vi "ELVIS III v1.1 Start AI Continuous.vi"(4 "Minimum (S/s)":dbl=1000.0, 5 "Sample Rate":dbl=1000.0 min=1000.0 max=1000000.0, 6 "Maximum (S/s)":dbl=1000000.0, 7 "Scaling Constants List":T1, 8 "error in (no error)":errorcluster, 10 "AI (Continuous) Channels List":T3, 11 "AI (Continuous) Ref In":T5) -> (0 "error out":errorcluster, 3 "AI (Continuous) Ref Out":T5)   [LabVIEW 2021]
uses:
  <vilib>/myRIO/Common/Instrument Driver Framework/Utilities/typedefs/myRIO v1.0 Reference.ctl
  <vilib>/myRIO/Common/Instrument Driver Framework/Utilities/typedefs/Generic FPGA Reference.ctl
  <vilib>/myRIO/Common/Instrument Driver Framework/ELVIS III v1.0/AI Continuous/typedefs/AI Continuous Channels List.ctl
  <vilib>/myRIO/Common/Instrument Driver Framework/ELVIS III v1.0/AI Continuous/typedefs/ELVIS III v1.0 AI Continuous Channels Enum.ctl
  <vilib>/myRIO/Common/Instrument Driver Framework/Utilities/typedefs/Analog Scaling Constants List.ctl
  <vilib>/myRIO/Common/Instrument Driver Framework/Utilities/typedefs/Analog Scaling Constants.ctl
  <vilib>/myRIO/Common/Instrument Driver Framework/ELVIS III v1.0/AI Block/typedefs/ELVIS III AI Block Channels FPGA Reference.ctl
  <vilib>/rvi/errors/niLvFpgaAdjustHostInterfaceError.vi
  <vilib>/rvi/interface/nirviReadWriteControl/nirviReadWriteControl.xnode
  <vilib>/rvi/interface/nirviMethod/nirviMethod.xnode
  <vilib>/rvi/errors/niLvFpgaMergeErrorWithErrorCode.vi
  <vilib>/rvi/interface/Simulation/niFpgaSimulationCallBeginRW.vi
  <vilib>/FPGAPlugInAG/Dynamic/niLvFpga_StartFifo_Dynamic.vi
  <vilib>/FPGAPlugInAG/Dynamic/niLvFpga_StopFifo_Dynamic.vi
  NiFpgaLv.dll
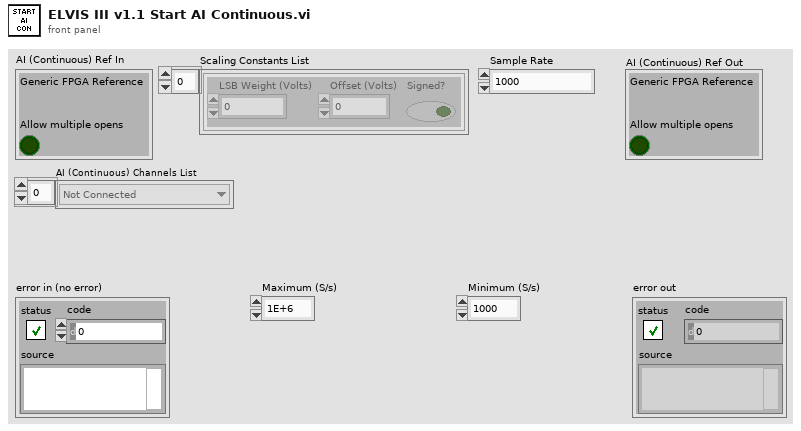
[diagram p1: front panel]
types:
  T1 = typedef "Analog Scaling Constants List.ctl" = T2[]
  T2 = typedef "Analog Scaling Constants.ctl" = cluster{"LSB Weight (Volts)":dbl, "Offset (Volts)":dbl, "Signed?":bool}
  T3 = typedef "AI Continuous Channels List.ctl" = T4[]
  T4 = typedef "ELVIS III v1.0 AI Continuous Channels Enum.ctl" = enum16{"Not Connected", "A/AI0 (Continuous)", "A/AI1 (Continuous)", "A/AI2 (Continuous)", "A/AI3 (Continuous)", "A/AI4 (Continuous)", "A/AI5 (Continuous)", "A/AI6 (Continuous)", "A/AI7 (Continuous)", "A/AI0 (DIFF Continuous)", "A/AI1 (DIFF Continuous)", "A/AI2 (DIFF Continuous)", "A/AI3 (DIFF Continuous)", "B/AI0 (Continuous)", "B/AI1 (Continuous)", "B/AI2 (Continuous)", "B/AI3 (Continuous)", "B/AI4 (Continuous)", "B/AI5 (Continuous)", "B/AI6 (Continuous)", "B/AI7 (Continuous)", "B/AI0 (DIFF Continuous)", "B/AI1 (DIFF Continuous)", "B/AI2 (DIFF Continuous)", "B/AI3 (DIFF Continuous)"}
  T5 = typedef "myRIO v1.0 Reference.ctl" = cluster{"Generic FPGA Reference":T6, "Allow multiple opens":bool}
  T6 = typedef "Generic FPGA Reference.ctl" = refnum<k20>
  T7 = typedef "ELVIS III AI Block Channels FPGA Reference.ctl" = refnum<k20>
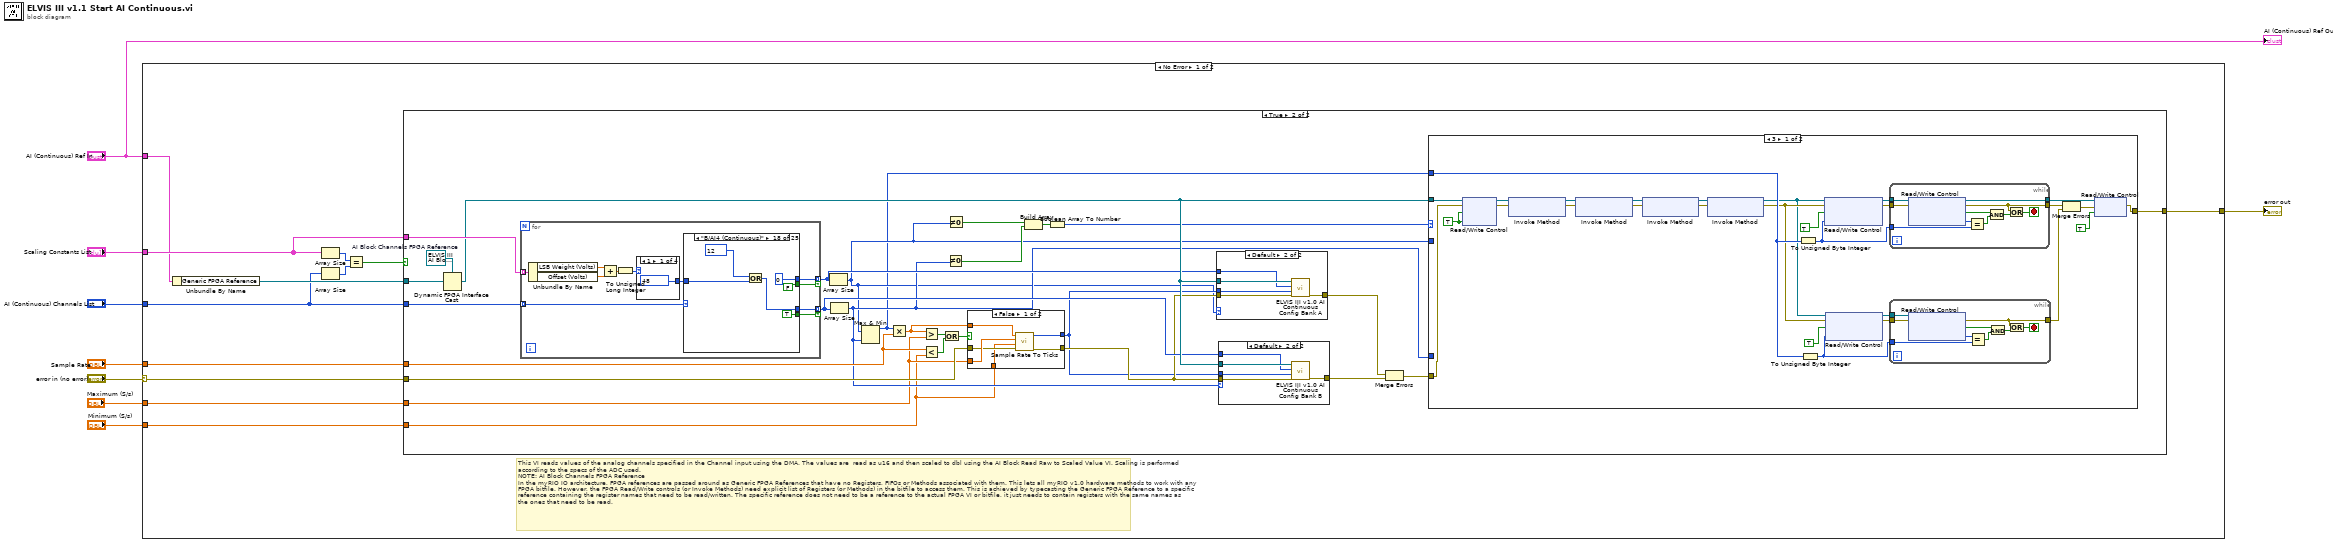
[diagram p0: block diagram]
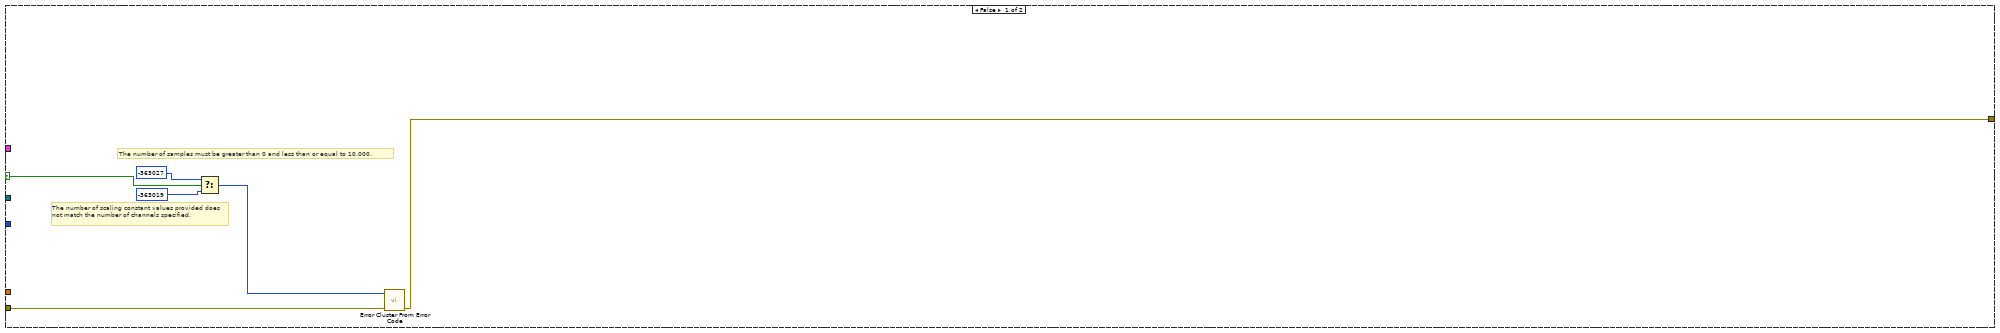
[diagram p2: hidden frame]
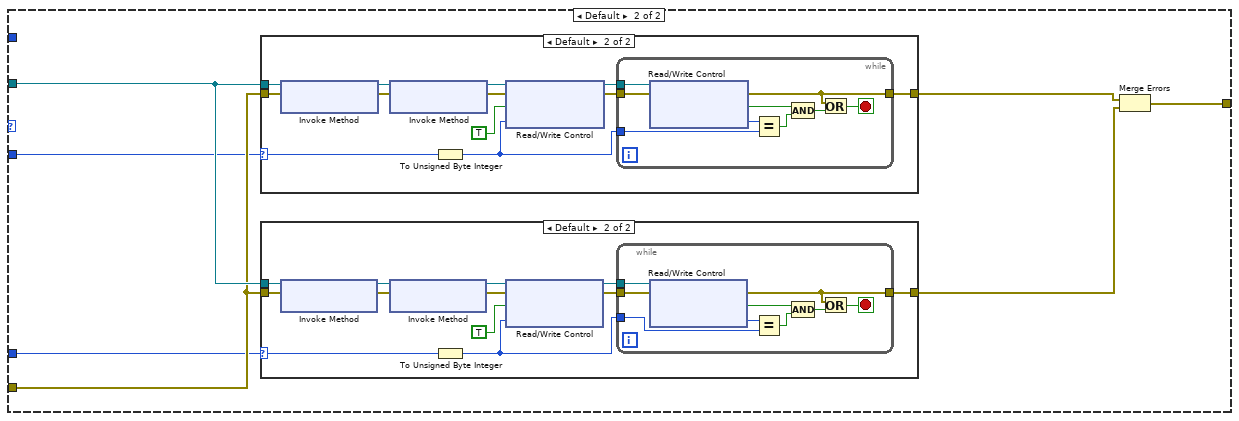
[diagram p3: hidden frame]
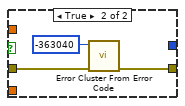
[diagram p6: hidden frame]
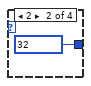
[diagram p7: hidden frame]
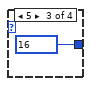
[diagram p8: hidden frame]
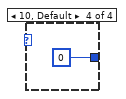
[diagram p9: hidden frame]
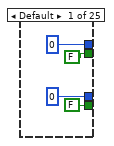
[diagram p10: hidden frame]
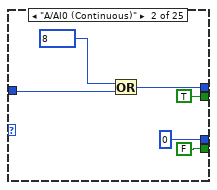
[diagram p11: hidden frame]
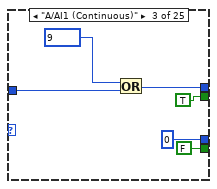
[diagram p12: hidden frame]
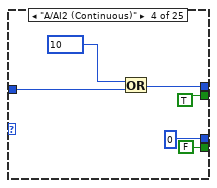
[diagram p13: hidden frame]
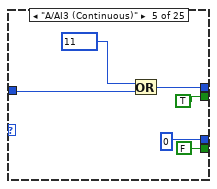
[diagram p14: hidden frame]
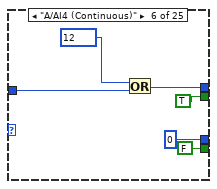
[diagram p15: hidden frame]
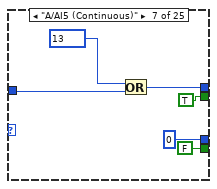
[diagram p16: hidden frame]
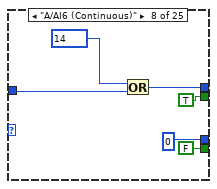
[diagram p17: hidden frame]
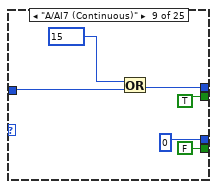
[diagram p18: hidden frame]
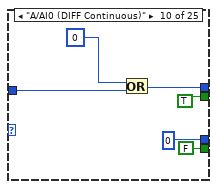
[diagram p19: hidden frame]
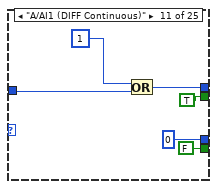
[diagram p20: hidden frame]
diagram:
  n1 = case shown="No Error" "error in (no error)" {
    selector: "error in (no error)" -> [w19 w337]
    tunnel: [w20 w337] -> w8
    tunnel: "Sample Rate" -> [w17 _]
    tunnel: "AI (Continuous) Ref In" -> [w11 _]
    tunnel: "Scaling Constants List" -> [w13 _]
    tunnel: "AI (Continuous) Channels List" -> [w12 _]
    tunnel: "Maximum (S/s)" -> [w10 _]
    tunnel: "Minimum (S/s)" -> [w9 _]
    frame No Error {
      # "This VI reads values of the analog channels specified in the Channel input using the DMA. The values are  read as u16 and then scaled to dbl using the AI Block Read Raw to Scaled Value VI. Scaling is performed according to the specs of the ADC used.\nNOTE: AI Block Channels FPGA Reference\nIn the myRIO IO architecture, FPGA references are passed around as Generic FPGA References that have no Registers, FIFOs or Methods associated with them. This lets all myRIO v1.0 hardware methods to work with any FPGA bitfile. However, the FPGA Read/Write controls (or Invoke Methods) need explicit list of Registers (or Methods) in the bitfile to access them. This is achieved by typecasting the Generic FPGA Reference to a specific reference containing the register names that need to be read/written. The specific reference does not need to be a reference to the actual FPGA VI or bitfile, it just needs to contain registers with the same names as the ones that need to be read."
      n2 = Unbundle By Name(w11) -> ("Generic FPGA Reference"=w18:T6)
      n3 = Array Size(array=w13) -> (size(s)=w15:i32)
      n4 = Array Size(array=w12) -> (size(s)=w16:i32)
      n5 = Equal?(x=w15, y=w16) -> (x = y?=w14:bool)
      n6 = case shown="True" w14 {
        selector: w14 -> [w23 _]
        tunnel: [w21 w54] -> w20
        tunnel: w19 -> [w22 w53]
        tunnel: w18 -> [_ w52]
        tunnel: w17 -> [_ w51]
        tunnel: w13 -> [_ w50]
        tunnel: w12 -> [_ w49]
        tunnel: w10 -> [_ w28]
        tunnel: w9 -> [_ w27]
        frame False {
          # "The number of samples must be greater than 0 and less than or equal to 10,000."
          # "The number of scaling constant values provided does not match the number of channels specified."
          n7 = Select(t=-363027 ("error code (0)"), s=w23, f=-363019 ("error code (0)")) -> (s? t:f=w26:i32)
          n8 = call <vilib>:"Error Cluster From Error Code.vi"("error in (no error)"=w22, "error code (0)"=w26) -> ("error out"=w21:errorcluster)  [unwired: 7 in]
        }
        frame True {
          w46 = T7 refnum  # AI Block Channels FPGA Reference
          n9 = Dynamic FPGA Interface Cast(Session In=w46, Type=w52) -> (Session Out=w48:T7)
          n10 = for {
            tunnel: w49 -> [w171] mode=indexing
            tunnel: w50 -> [w163] mode=indexing
            tunnel: [w172] -> w43 mode=indexing if=w170
            tunnel: [w169] -> w42 mode=indexing if=w168
            n11 = Unbundle By Name(w163) -> ("LSB Weight (Volts)"=w165:dbl, "Offset (Volts)"=w164:dbl)
            n12 = Add(x=w165, y=w164) -> (x+y=w166:dbl)
            n13 = To Unsigned Long Integer(number=w166) -> (unsigned 32bit integer=w167:u32)
            n14 = case shown="1" w167 {
              tunnel: [u8 48 u8 32 u8 16 u8 0] -> w162
              frame 1 {
              }
              frame 2 {
              }
              frame 5 {
              }
              frame 10, Default {
              }
            }
            n15 = case shown="\"B/AI4 (Continuous)\"" w171 {
              tunnel: [u8 0 w182 w188 w194 w200 w206 w212 w218 w224 w230 w236 w242 w248 u8 0 u8 0 u8 0 u8 0 u8 0 u8 0 u8 0 u8 0 u8 0 u8 0 u8 0 u8 0] -> w172
              tunnel: [FALSE TRUE TRUE TRUE TRUE TRUE TRUE TRUE TRUE TRUE TRUE TRUE TRUE FALSE FALSE FALSE FALSE FALSE FALSE FALSE FALSE FALSE FALSE FALSE FALSE] -> w170
              tunnel: [u8 0 u8 0 u8 0 u8 0 u8 0 u8 0 u8 0 u8 0 u8 0 u8 0 u8 0 u8 0 u8 0 w254 w260 w266 w272 w278 w284 w290 w296 w302 w308 w314 w320] -> w169
              tunnel: [FALSE FALSE FALSE FALSE FALSE FALSE FALSE FALSE FALSE FALSE FALSE FALSE FALSE TRUE TRUE TRUE TRUE TRUE TRUE TRUE TRUE TRUE TRUE TRUE TRUE] -> w168
              tunnel: w162 -> [_ w181 w187 w193 w199 w205 w211 w217 w223 w229 w235 w241 w247 w253 w259 w265 w271 w277 w283 w289 w295 w301 w307 w313 w319]
              frame Default {
              }
              frame "A/AI0 (Continuous)" {
                n16 = Or(x=u8 8, y=w181) -> (x .or. y?=w182:u8)
              }
              frame "A/AI1 (Continuous)" {
                n17 = Or(x=u8 9, y=w187) -> (x .or. y?=w188:u8)
              }
              frame "A/AI2 (Continuous)" {
                n18 = Or(x=u8 10, y=w193) -> (x .or. y?=w194:u8)
              }
              frame "A/AI3 (Continuous)" {
                n19 = Or(x=u8 11, y=w199) -> (x .or. y?=w200:u8)
              }
              frame "A/AI4 (Continuous)" {
                n20 = Or(x=u8 12, y=w205) -> (x .or. y?=w206:u8)
              }
              frame "A/AI5 (Continuous)" {
                n21 = Or(x=u8 13, y=w211) -> (x .or. y?=w212:u8)
              }
              frame "A/AI6 (Continuous)" {
                n22 = Or(x=u8 14, y=w217) -> (x .or. y?=w218:u8)
              }
              frame "A/AI7 (Continuous)" {
                n23 = Or(x=u8 15, y=w223) -> (x .or. y?=w224:u8)
              }
              frame "A/AI0 (DIFF Continuous)" {
                n24 = Or(x=u8 0, y=w229) -> (x .or. y?=w230:u8)
              }
              frame "A/AI1 (DIFF Continuous)" {
                n25 = Or(x=u8 1, y=w235) -> (x .or. y?=w236:u8)
              }
              frame "A/AI2 (DIFF Continuous)" {
                n26 = Or(x=u8 2, y=w241) -> (x .or. y?=w242:u8)
              }
              frame "A/AI3 (DIFF Continuous)" {
                n27 = Or(x=u8 3, y=w247) -> (x .or. y?=w248:u8)
              }
              frame "B/AI0 (Continuous)" {
                n28 = Or(x=u8 8, y=w253) -> (x .or. y?=w254:u8)
              }
              frame "B/AI1 (Continuous)" {
                n29 = Or(x=u8 9, y=w259) -> (x .or. y?=w260:u8)
              }
              frame "B/AI2 (Continuous)" {
                n30 = Or(x=u8 10, y=w265) -> (x .or. y?=w266:u8)
              }
              frame "B/AI3 (Continuous)" {
                n31 = Or(x=u8 11, y=w271) -> (x .or. y?=w272:u8)
              }
              frame "B/AI4 (Continuous)" {
                n32 = Or(x=u8 12, y=w277) -> (x .or. y?=w278:u8)
              }
              frame "B/AI5 (Continuous)" {
                n33 = Or(x=u8 13, y=w283) -> (x .or. y?=w284:u8)
              }
              frame "B/AI6 (Continuous)" {
                n34 = Or(x=u8 14, y=w289) -> (x .or. y?=w290:u8)
              }
              frame "B/AI7 (Continuous)" {
                n35 = Or(x=u8 15, y=w295) -> (x .or. y?=w296:u8)
              }
              frame "B/AI0 (DIFF Continuous)" {
                n36 = Or(x=u8 0, y=w301) -> (x .or. y?=w302:u8)
              }
              frame "B/AI1 (DIFF Continuous)" {
                n37 = Or(x=u8 1, y=w307) -> (x .or. y?=w308:u8)
              }
              frame "B/AI2 (DIFF Continuous)" {
                n38 = Or(x=u8 2, y=w313) -> (x .or. y?=w314:u8)
              }
              frame "B/AI3 (DIFF Continuous)" {
                n39 = Or(x=u8 3, y=w319) -> (x .or. y?=w320:u8)
              }
            }
          }
          n40 = Array Size(array=w43) -> (size(s)=w30:i32)
          n41 = Array Size(array=w42) -> (size(s)=w35:i32)
          n42 = Max & Min(x=w30, y=w35) -> (max(x,y)=w29:i32)  [unwired: 1 out]
          n43 = Multiply(x=w29, y=w51) -> (x*y=w36:dbl)
          n44 = Greater?(x=w36, y=w28) -> (0:w41:bool)
          n45 = Less?(x=w51, y=w27) -> (x < y?=w40:bool)
          n46 = Or(x=w41, y=w40) -> (x .or. y?=w39:bool)
          n47 = Not Equal To 0?(x=w35) -> (x != 0?=w32:bool)
          n48 = Not Equal To 0?(x=w30) -> (x != 0?=w33:bool)
          n49 = case shown="False" w39 {
            tunnel: w53 -> [w154 w160]
            tunnel: [w157 w159] -> w38
            tunnel: [w158 _] -> w37
            tunnel: w36 -> [w156 _]
            tunnel: w28 -> [w155 _]
            tunnel: w27 -> [w153 _]
            frame False {
              n50 = call <vilib>:"Sample Rate To Ticks.vi"("error in (no error)"=w154, "Minimum (S/s)"=w153, "Maximum (S/s)"=w155, "Sample Rate (S/s)"=w156) -> ("error out"=w157:errorcluster, "Count (tick/s)"=w158:u32)  [unwired: 5 in, 1 out]
            }
            frame True {
              n51 = call <vilib>:"Error Cluster From Error Code.vi"("error in (no error)"=w160, "error code (0)"=-363040) -> ("error out"=w159:errorcluster)  [unwired: 7 in]
            }
          }
          n52 = Build Array(w33, w32) -> (w34:bool[])
          n53 = Boolean Array To Number(Boolean array=w34) -> (number=w31:u32)
          n54 = case shown="Default" w30 {
            tunnel: w48 -> [_ w336]
            tunnel: w37 -> [_ w335]
            tunnel: w38 -> [w331 w334]
            tunnel: [w331 w333] -> w45
            tunnel: w43 -> [_ w332]
            frame 0 {
            }
            frame Default {
              n55 = call <vilib>:"ELVIS III v1.0 AI Continuous Config Bank A.vi"("AI (Continuous) Channels FPGA Reference"=w336, "Bank Config"=w332, "Count (tick/s)"=w335, "error in (no error)"=w334) -> ("error out"=w333:errorcluster)  [unwired: 6 in]
            }
          }
          n56 = case shown="Default" w35 {
            tunnel: w48 -> [_ w330]
            tunnel: w37 -> [_ w329]
            tunnel: w38 -> [w325 w328]
            tunnel: [w325 w327] -> w44
            tunnel: w42 -> [_ w326]
            frame 0 {
            }
            frame Default {
              n57 = call <vilib>:"ELVIS III v1.0 AI Continuous Config Bank B.vi"("AI (Continuous) Channels FPGA Reference"=w330, "Bank Config"=w326, "Count (tick/s)"=w329, "error in (no error)"=w328) -> ("error out"=w327:errorcluster)  [unwired: 6 in]
            }
          }
          n58 = Merge Errors(w45, w44) -> (w47:errorcluster)
          n59 = case shown="3" w31 {
            tunnel: [w71 w108] -> w54
            tunnel: w48 -> [w57 w107]
            tunnel: w47 -> [w59 w106]
            tunnel: w30 -> [_ w103]
            tunnel: w35 -> [_ w102]
            tunnel: w29 -> [w70 _]
            frame 3 {
              w55 = TRUE ("A.SYNC")
              n60 = xnode "Read/Write Control"("FPGA VI Reference In"=w57, "error in"=w59, "A.SYNC"=w55, "B.SYNC"=w55) -> ("FPGA VI Reference Out"=w68:T7, "error out"=w69:errorcluster)
              n61 = xnode "Invoke Method"("FPGA VI Reference In"=w68, "error in"=w69) -> ("FPGA VI Reference Out"=w62:T7, "error out"=w63:errorcluster)
              n62 = xnode "Invoke Method"("FPGA VI Reference In"=w62, "error in"=w63) -> ("FPGA VI Reference Out"=w66:T7, "error out"=w67:errorcluster)
              n63 = xnode "Invoke Method"("FPGA VI Reference In"=w66, "error in"=w67) -> ("FPGA VI Reference Out"=w64:T7, "error out"=w65:errorcluster)
              n64 = xnode "Invoke Method"("FPGA VI Reference In"=w64, "error in"=w65) -> ("FPGA VI Reference Out"=w56:T7, "error out"=w58:errorcluster)
              n65 = To Unsigned Byte Integer(number=w70) -> (unsigned 8bit integer=w79:u8)
              n66 = To Unsigned Byte Integer(number=w70) -> (unsigned 8bit integer=w78:u8)
              n67 = xnode "Read/Write Control"("FPGA VI Reference In"=w56, "error in"=w58, "AI.A.DMA_ENA"=TRUE, "AI.A.CNT"=w79) -> ("FPGA VI Reference Out"=w81:T7, "error out"=w82:errorcluster)
              n68 = xnode "Read/Write Control"("FPGA VI Reference In"=w56, "error in"=w58, "AI.B.DMA_ENA"=TRUE, "AI.B.CNT"=w78) -> ("FPGA VI Reference Out"=w76:T7, "error out"=w75:errorcluster)
              n69 = while {
                tunnel: w82 -> [w101]
                tunnel: w81 -> [w100]
                tunnel: [w95] -> w74
                tunnel: w79 -> [w99]
                tunnel: [w92] -> w60
                stop <- w93 stop-if-true
                n70 = xnode "Read/Write Control"("FPGA VI Reference In"=w100, "error in"=w101) -> ("FPGA VI Reference Out"=w92:T7, "error out"=w95:errorcluster, "AI.A.DMA_ENA"=w97:bool, "AI.A.CNT"=w98:u8)
                n71 = Equal?(x=w98, y=w99) -> (x = y?=w96:bool)
                n72 = Compound Arithmetic op=AND(w97, w96) -> (w94:bool)
                n73 = Or(x=w95, y=w94) -> (x .or. y?=w93:bool)
              }
              n74 = while {
                tunnel: w75 -> [w91]
                tunnel: w76 -> [w90]
                tunnel: [w85] -> w73
                tunnel: w78 -> [w89]
                stop <- w83 stop-if-true
                n75 = xnode "Read/Write Control"("FPGA VI Reference In"=w90, "error in"=w91) -> ("error out"=w85:errorcluster, "AI.B.DMA_ENA"=w87:bool, "AI.B.CNT"=w88:u8)  [unwired: 1 out]
                n76 = Equal?(x=w88, y=w89) -> (x = y?=w86:bool)
                n77 = Compound Arithmetic op=AND(w87, w86) -> (w84:bool)
                n78 = Or(x=w85, y=w84) -> (x .or. y?=w83:bool)
              }
              n79 = Merge Errors(w74, w73) -> (w61:errorcluster)
              n80 = xnode "Read/Write Control"("FPGA VI Reference In"=w60, "error in"=w61, "SYNC"=TRUE) -> ("error out"=w71:errorcluster)  [unwired: 1 out]
            }
            frame Default {
              n81 = case shown="Default" w103 {
                selector: w103 -> [_ w115]
                tunnel: w107 -> [_ w114]
                tunnel: w106 -> [w109 w113]
                tunnel: [w109 w112] -> w105
                frame 0 {
                }
                frame Default {
                  n82 = xnode "Invoke Method"("FPGA VI Reference In"=w114, "error in"=w113) -> ("FPGA VI Reference Out"=w121:T7, "error out"=w120:errorcluster)
                  n83 = xnode "Invoke Method"("FPGA VI Reference In"=w121, "error in"=w120) -> ("FPGA VI Reference Out"=w119:T7, "error out"=w118:errorcluster)
                  n84 = To Unsigned Byte Integer(number=w115) -> (unsigned 8bit integer=w111:u8)
                  n85 = xnode "Read/Write Control"("FPGA VI Reference In"=w119, "error in"=w118, "AI.A.DMA_ENA"=TRUE, "AI.A.CNT"=w111) -> ("FPGA VI Reference Out"=w116:T7, "error out"=w117:errorcluster)
                  n86 = while {
                    tunnel: w117 -> [w130]
                    tunnel: w116 -> [w129]
                    tunnel: [w124] -> w112
                    tunnel: w111 -> [w128]
                    stop <- w122 stop-if-true
                    n87 = xnode "Read/Write Control"("FPGA VI Reference In"=w129, "error in"=w130) -> ("error out"=w124:errorcluster, "AI.A.DMA_ENA"=w126:bool, "AI.A.CNT"=w127:u8)  [unwired: 1 out]
                    n88 = Equal?(x=w127, y=w128) -> (x = y?=w125:bool)
                    n89 = Compound Arithmetic op=AND(w126, w125) -> (w123:bool)
                    n90 = Or(x=w124, y=w123) -> (x .or. y?=w122:bool)
                  }
                }
              }
              n91 = case shown="Default" w102 {
                selector: w102 -> [_ w135]
                tunnel: w107 -> [_ w137]
                tunnel: w106 -> [w131 w136]
                tunnel: [w131 w134] -> w104
                frame 0 {
                }
                frame Default {
                  n92 = xnode "Invoke Method"("FPGA VI Reference In"=w137, "error in"=w136) -> ("FPGA VI Reference Out"=w143:T7, "error out"=w142:errorcluster)
                  n93 = xnode "Invoke Method"("FPGA VI Reference In"=w143, "error in"=w142) -> ("FPGA VI Reference Out"=w141:T7, "error out"=w140:errorcluster)
                  n94 = To Unsigned Byte Integer(number=w135) -> (unsigned 8bit integer=w133:u8)
                  n95 = xnode "Read/Write Control"("FPGA VI Reference In"=w141, "error in"=w140, "AI.B.DMA_ENA"=TRUE, "AI.B.CNT"=w133) -> ("FPGA VI Reference Out"=w138:T7, "error out"=w139:errorcluster)
                  n96 = while {
                    tunnel: w139 -> [w152]
                    tunnel: w138 -> [w151]
                    tunnel: [w149] -> w134
                    tunnel: w133 -> [w150]
                    stop <- w148 stop-if-true
                    n97 = xnode "Read/Write Control"("FPGA VI Reference In"=w151, "error in"=w152) -> ("error out"=w149:errorcluster, "AI.B.DMA_ENA"=w144:bool, "AI.B.CNT"=w147:u8)  [unwired: 1 out]
                    n98 = Equal?(x=w147, y=w150) -> (x = y?=w146:bool)
                    n99 = Compound Arithmetic op=AND(w144, w146) -> (w145:bool)
                    n100 = Or(x=w149, y=w145) -> (x .or. y?=w148:bool)
                  }
                }
              }
              n101 = Merge Errors(w105, w104) -> (w108:errorcluster)
            }
          }
        }
      }
    }
    frame Error {
    }
  }
  "error out" <- w8
  "AI (Continuous) Ref Out" <- "AI (Continuous) Ref In"
